vi "SwerveModifyDriveCommand.vi"(1 "Azimuth Error (deg)":dbl, 2 "Flip Drive Command":bool, 3 "Raw Drive Command (ul)":dbl) -> (0 "Modified Drive Command (ul)":dbl format="%.3f")   [LabVIEW 2019]
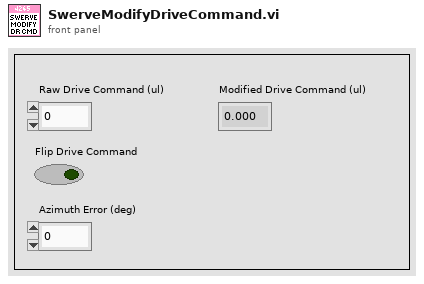
[diagram p1: front panel]
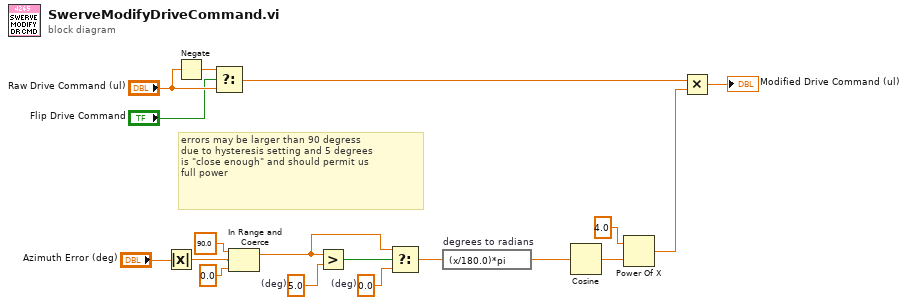
[diagram p0: block diagram]
diagram:
  w4 = 0.0  # (deg)
  w2 = 5.0  # (deg)
  # "errors may be larger than 90 degress\ndue to hysteresis setting and 5 degrees\nis \"close enough\" and should permit us\nfull power"
  n1 = Absolute Value(x="Azimuth Error (deg)") -> (abs(x)=w7:dbl)
  n2 = Negate(x="Raw Drive Command (ul)") -> (-x=w17:dbl)
  n3 = Select(t=w17, s="Flip Drive Command", f="Raw Drive Command (ul)") -> (s? t:f=w15:dbl)
  n4 = In Range and Coerce(upper limit=90.0, x=w7, lower limit=0.0) -> (coerced(x)=w3:dbl)  [unwired: 1 out]
  n5 = Greater?(x=w3, y=w2) -> (0:w5:bool)
  n6 = Select(t=w3, s=w5, f=w4) -> (s? t:f=w1:dbl)
  n7 = expression code="(x/180.0)*pi" "degrees to radians"(w1) -> (w6:dbl)
  n8 = Cosine(x=w6) -> (cos(x)=w12:dbl)
  n9 = Power Of X(1:w12, 2:4.0 ("y")) -> (0:w10:dbl)
  n10 = Multiply(x=w15, y=w10) -> (x*y=→"Modified Drive Command (ul)":dbl)
